vi "Coordinates to Array Index.vi"(8 "error in (no error)":errorcluster, 10 "Coordinates":cluster{"Horizontal":i32, "Vertical":i32}, 11 "Array ref":refnum<vi>) -> (0 "error out":errorcluster, 2 "Column Index":i32, 3 "Row Index":i32, 5 "Vertical In Range?":bool, 7 "Horizontal In Range?":bool)   [LabVIEW 2017, in "Front Panel Publisher.lvlib" / "Web Front Panel.lvclass"]
doc: "Given a reference to a 1-D or 2-D array, and screen coordinates,\nreturn the index of the element at that location.\nTwo values are returned: col index is valid for horizontal arrays, and row index is valid for vertical arrays, both are valid for 2-D arrays."
uses:
  Web Front Panel.lvclass
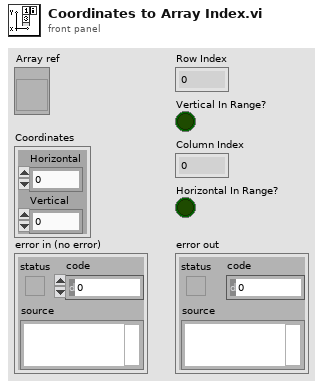
[diagram p1: front panel]
types:
  T1 = typedef "LVRectTypeDef.ctl" = cluster{"Left":i16, "Top":i16, "Right":i16, "Bottom":i16}
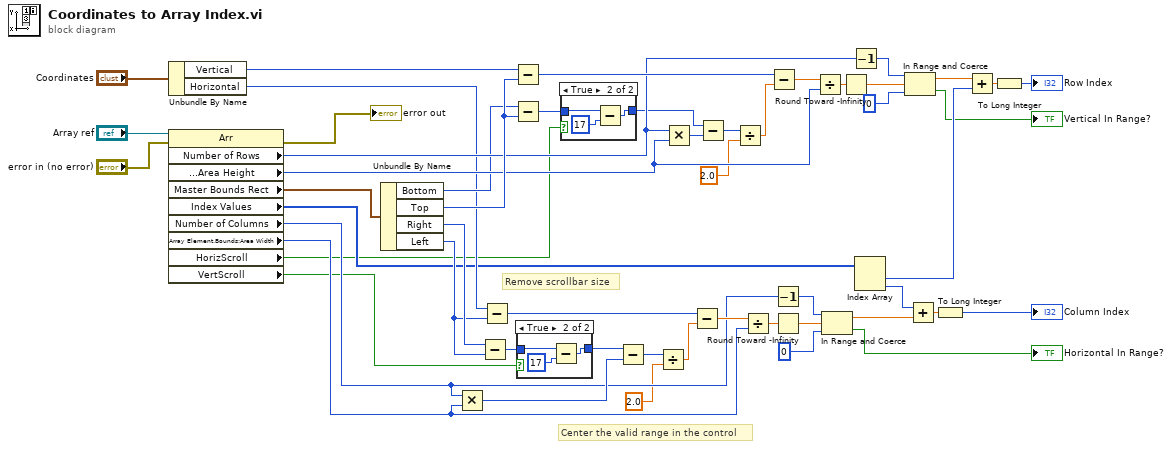
[diagram p0: block diagram]
diagram:
  # "Remove scrollbar size"
  # "Center the valid range in the control"
  n1 = Unbundle By Name("Coordinates") -> ("Vertical"=w47:i32, "Horizontal"=w13:i32)
  n2 = property on="Property Node" class="Arr"(reference="Array ref", error in="error in (no error)") -> (error out=→"error out":errorcluster, "Number of Rows"=w17:u32, "Array Element.Bounds:Area Height"=w23:u32, "Master Bounds Rect"=w16:T1, "Index Values"=w12:u32[], "Number of Columns"=w20:u32, "Array Element.Bounds:Area Width"=w19:u32, "HorizScroll"=w2:bool, "VertScroll"=w5:bool)  [unwired: 1 out]
  n3 = Unbundle By Name(w16) -> ("Bottom"=w15:i16, "Top"=w24:i16, "Right"=w21:i16, "Left"=w14:i16)
  n4 = Multiply(x=w20, y=w19) -> (x*y=w36:u32)
  n5 = Subtract(x=w21, y=w14) -> (x-y=w6:i16)
  n6 = Subtract(x=w13, y=w14) -> (x-y=w34:i32)
  n7 = Subtract(x=w47, y=w24) -> (x-y=w29:i32)
  n8 = Subtract(x=w15, y=w24) -> (x-y=w3:i16)
  n9 = case shown="True" w5 {
    tunnel: w6 -> [w53 w56]
    tunnel: [w53 w55] -> w4
    frame False {
    }
    frame True {
      n10 = Subtract(x=w56, y=i16 17) -> (x-y=w55:i16)
    }
  }
  n11 = case shown="True" w2 {
    tunnel: w3 -> [w57 w60]
    tunnel: [w57 w59] -> w1
    frame False {
    }
    frame True {
      n12 = Subtract(x=w60, y=i16 17) -> (x-y=w59:i16)
    }
  }
  n13 = Subtract(x=w4, y=w36) -> (x-y=w9:u32)
  n14 = Divide(x=w9, y=2.0) -> (x/y=w35:dbl)
  n15 = Multiply(x=w17, y=w23) -> (x*y=w31:u32)
  n16 = Subtract(x=w34, y=w35) -> (x-y=w33:dbl)
  n17 = Subtract(x=w1, y=w31) -> (x-y=w32:u32)
  n18 = Divide(x=w32, y=2.0) -> (x/y=w30:dbl)
  n19 = Divide(x=w33, y=w19) -> (x/y=w39:dbl)
  n20 = Subtract(x=w29, y=w30) -> (x-y=w28:dbl)
  n21 = Decrement(x=w20) -> (x-1=w44:u32)
  n22 = Round Toward -Infinity(1:w39) -> (0:w26:dbl)
  n23 = Divide(x=w28, y=w23) -> (x/y=w40:dbl)
  n24 = In Range and Coerce(upper limit=w44, x=w26, lower limit=u32 0) -> (coerced(x)=w11:dbl, In Range?=→"Horizontal In Range?":bool)
  n25 = Round Toward -Infinity(1:w40) -> (0:w27:dbl)
  n26 = Decrement(x=w17) -> (x-1=w49:u32)
  n27 = Index Array(array=w12) -> (element #1=w51:u32, element #2=w10:u32)  [unwired: 2 in]
  n28 = In Range and Coerce(upper limit=w49, x=w27, lower limit=u32 0) -> (coerced(x)=w52:dbl, In Range?=→"Vertical In Range?":bool)
  n29 = Add(x=w10, y=w11) -> (x+y=w45:dbl)
  n30 = To Long Integer(number=w45) -> (32bit integer=→"Column Index":i32)
  n31 = Add(x=w52, y=w51) -> (x+y=w50:dbl)
  n32 = To Long Integer(number=w50) -> (32bit integer=→"Row Index":i32)
